vi "Stop Measurements Command.vi"(8 "error in (no error)":errorcluster, 10 "Measurement Controller":string, 11 "Application Controller in":refnum<class "Application Controller.lvclass">) -> (0 "error out":errorcluster, 3 "Application Controller out":refnum<class "Application Controller.lvclass">)   [LabVIEW 2021, in "Application Controller.lvclass"]
uses:
  Controllers/Application Controller/Application Controller.lvclass
  Controllers/Process Controller/Request type.ctl
  Controllers/Process Controller Messages/Stop Measurements Msg/Stop Measurements Msg.lvclass/Stop Measurements Msg.ctl
  <vilib>/ActorFramework/Message Enqueuer/Message Enqueuer.lvclass/Message Enqueuer.ctl
  <vilib>/ActorFramework/Message Enqueuer/Enqueue.vi
  Controllers/Process Controller Messages/Stop Measurements Msg/Stop Measurements Msg.lvclass
  C:/Program Files/National Instruments/LabVIEW 2021/vi.lib/ActorFramework/Message/Message.lvclass
  <vilib>/ActorFramework/Message Priority Queue/Priority Enqueue.vi
  Controllers/Application Controller/Application Controller.lvclass/Application Controller.ctl
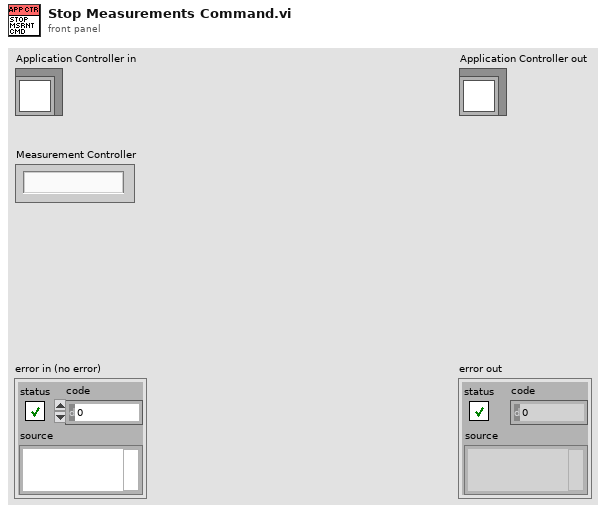
[diagram p1: front panel]
types:
  T1 = typedef "Request type.ctl" = enum16{"Process complete", "User command", "Auto-restart", "Error"}
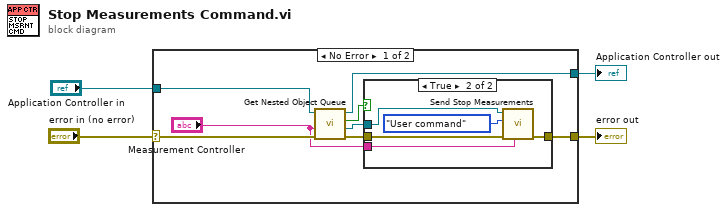
[diagram p0: block diagram]
diagram:
  n1 = case shown="No Error" "error in (no error)" {
    selector: "error in (no error)" -> [w8 w20]
    tunnel: [w6 w20] -> w3
    tunnel: [w10 w19] -> w1
    tunnel: "Application Controller in" -> [w11 w19]
    frame No Error {
      n2 = call-dynamic "Get Nested Object Queue.vi"("error in (no error)"=w8, "Name"="Measurement Controller", "Measure Object in"=w11) -> ("error out"=w7:errorcluster, "Object Enqueuer"=w12:refnum<class "Message Enqueuer.lvclass">, "Found?"=w9:bool, "Measure Object out"=w10:refnum<class "Application Controller.lvclass">)  [unwired: 5 in]
      n3 = case shown="True" w9 {
        tunnel: w12 -> [_ w18]
        tunnel: w7 -> [w13 w17]
        tunnel: [w13 w16] -> w6
        tunnel: "Measurement Controller" -> [_ w14]
        frame False {
        }
        frame True {
          n4 = call "Send Stop Measurements.vi"("Controller name"=w14, "error in (no error)"=w17, "Request type"=Request_type."User command", "Message Enqueuer"=w18) -> ("error out"=w16:errorcluster)  [unwired: 6 in, 1 out]
        }
      }
    }
    frame Error {
    }
  }
  "error out" <- w3
  "Application Controller out" <- w1
